vi "Get Vars From Function Node.vi"(11 "Refnum in":refnum<k20>) -> (3 "Variables":map{string, T1}(c390))   [LabVIEW 2021]
uses:
  Node.ctl
  Variable Type.ctl
  <vilib>/xml/NI_XML.lvlib
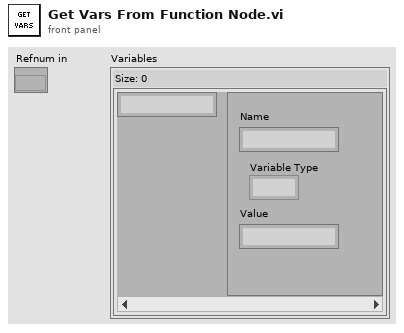
[diagram p1: front panel]
types:
  T1 = typedef "Node.ctl" = cluster{"Name":string, "Variable Type":T2, "Value":string}
  T2 = typedef "Variable Type.ctl" = enum16{"INT", "DOUBLE", "STRING"}
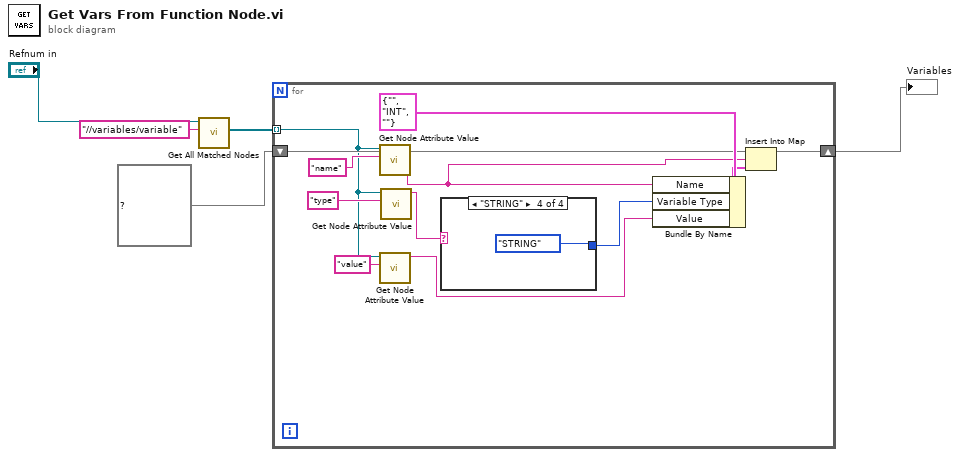
[diagram p0: block diagram]
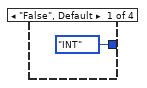
[diagram p2: hidden frame]
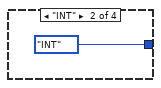
[diagram p3: hidden frame]
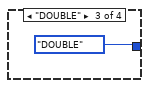
[diagram p4: hidden frame]
diagram:
  n1 = call <vilib>:"Get All Matched Nodes.vi"("XPath expression"="//variables/variable", "node in"="Refnum in") -> ("node result array"=w3:refnum<k20>[])  [unwired: 7 in, 2 out]
  n2 = for {
    tunnel: w3 -> [w8] mode=indexing
    shift-right: [w15] -> w5
    shift-left: map{string, T1} {} ("Variables") -> [w16]
    n3 = call "Get Node Attribute Value.vi"("Attribute Name"="name", "Refnum in"=w8) -> ("Value"=w14:string)  [unwired: 9 in]
    n4 = call "Get Node Attribute Value.vi"("Attribute Name"="value", "Refnum in"=w8) -> ("Value"=w6:string)  [unwired: 9 in]
    n5 = call "Get Node Attribute Value.vi"("Attribute Name"="type", "Refnum in"=w8) -> ("Value"=w10:string)  [unwired: 9 in]
    n6 = case shown="\"STRING\"" w10 {
      tunnel: [Variable_Type."INT" ("Variable Type") Variable_Type."INT" ("Variable Type") Variable_Type."DOUBLE" ("Variable Type") Variable_Type."STRING" ("Variable Type")] -> w9
      frame "False", Default {
      }
      frame "INT" {
      }
      frame "DOUBLE" {
      }
      frame "STRING" {
      }
    }
    n7 = Bundle By Name(cluster=T1 {"Name"="", "Variable Type"=enum."INT", "Value"=""} ("Variable"), "Name"=w14, "Variable Type"=w9, "Value"=w6) -> (w13:T1)
    n8 = Insert Into Map(map in=w16, key=w14, value=w13) -> (map out=w15:map{string, T1})  [unwired: 2 out]
  }
  "Variables" <- w5
